vi "Set References.vi"(8 "error in (no error)":errorcluster, 9 "Status References":refnum<vi>[](array[refnum]), 10 "Serial References":refnum<vi>[](array[refnum]), 11 "Template Properties in":refnum<class "App Properties.lvclass">) -> (0 "error out":errorcluster, 3 "Template Properties out":refnum<class "App Properties.lvclass">)   [LabVIEW 2017, in "Application.lvlib" / "App Properties.lvclass"]
uses:
  App Properties.lvclass
  UUT Reference -- Cluster.ctl
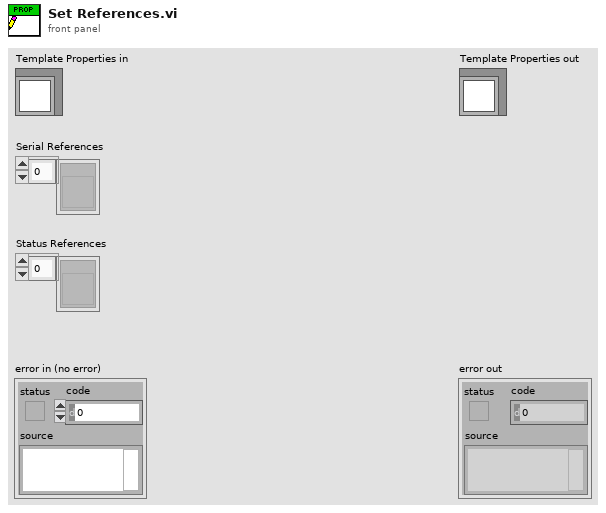
[diagram p1: front panel]
types:
  T1 = typedef "Application.lvlib/App Properties.lvclass/UUT Reference -- Cluster.ctl" = cluster{"Serial Number Reference":refnum<vi>, "Status Message Reference":refnum<vi>}
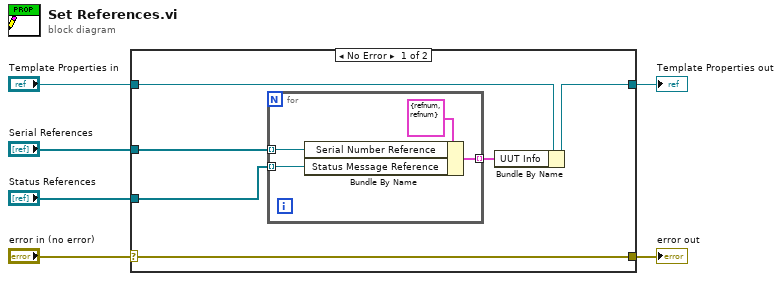
[diagram p0: block diagram]
diagram:
  n1 = case shown="No Error" "error in (no error)" {
    selector: "error in (no error)" -> [w12 w17]
    tunnel: [w12 w17] -> w5
    tunnel: [w10 w18] -> w3
    tunnel: "Template Properties in" -> [w11 w18]
    tunnel: "Serial References" -> [w9 _]
    tunnel: "Status References" -> [w8 _]
    frame No Error {
      n2 = for {
        tunnel: w9 -> [w15] mode=indexing
        tunnel: w8 -> [w14] mode=indexing
        tunnel: [w13] -> w7 mode=indexing
        n3 = Bundle By Name(cluster=T1 {"Serial Number Reference"=refnum, "Status Message Reference"=refnum} ("UUT Information"), "Serial Number Reference"=w15, "Status Message Reference"=w14) -> (w13:T1)
      }
      n4 = Bundle By Name(cluster=w11, "UUT Info"=w7) -> (w10:refnum<class "App Properties.lvclass">)
    }
    frame Error {
    }
  }
  "error out" <- w5
  "Template Properties out" <- w3
